vi "Log Plugin Errors.vi"(8 "error in (no error)":errorcluster, 11 "Full Plugin Array":T1[](array[typedef])) -> (0 "error out":errorcluster)   [LabVIEW 2020, in "RxnRover.lvlib" / "Plugin Manager.lvlib"]
doc: "This VI logs errors within invalid RxnRover plugins in a .txt file located at : \nwith the format;\n[Time RTC 3339] [Plugin name] Error : (error message) \n[Time RTC 3339] [Plugin name] Error : (error message) \n[Time RTC 3339] [Plugin name] Error : (error message) \n. . .\n\nIf there are no errors present, or invalid plugins, a .txt log file will not be created.\nlog file is overwritten at the standard path each time Load Plugins.vi is called (It does not create an additional log file)\nErrors are generated within the Read Configuration File .vi and sorted as invalid plugins within the Filter Invalid Plugins.vi\n\nCreated 5/20/2025 - Labview 2020\nRxnRover"
uses:
  Plugin Manager.lvlib
  Plugin Details.ctl
  Plugin Servers/Controller/Controller Type.ctl
  Plugin Types.ctl
  Config Error.ctl
  logging/logging.lvlib
  Plugin Servers/Controller/Generic Plugin.lvclass
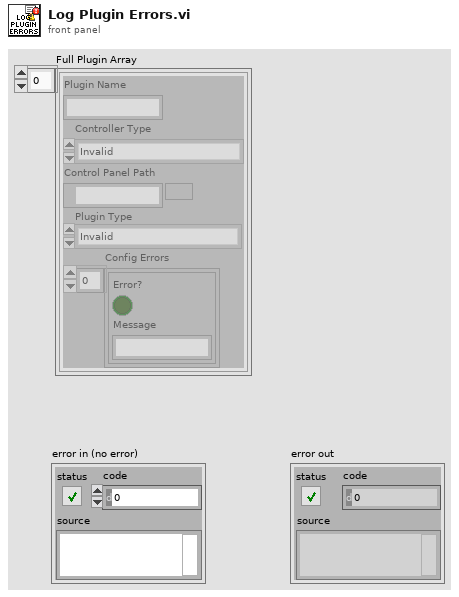
[diagram p1: front panel]
types:
  T1 = typedef "RxnRover.lvlib/Plugin Manager.lvlib/Plugin Details.ctl" = cluster{"Plugin Name":string, "Controller Type":T2, "Control Panel Path":path, "Plugin Type":T3, "Config Errors":T4[]}
  T2 = typedef "RxnRover.lvlib/Generic Plugin.lvclass/Controller Type.ctl" = enum16{"Invalid", "Temperature Controller", "Pump Controller", "Syringe Pump", "Generic Optimizer", "LC Parser", "Passive Hardware"}
  T3 = typedef "RxnRover.lvlib/Plugin Manager.lvlib/Plugin Types.ctl" = enum16{"Invalid", "Optimizer", "Analyzer", "Hardware"}
  T4 = typedef "RxnRover.lvlib/Plugin Manager.lvlib/Config Error.ctl" = cluster{"Error?":bool, "Message":string}
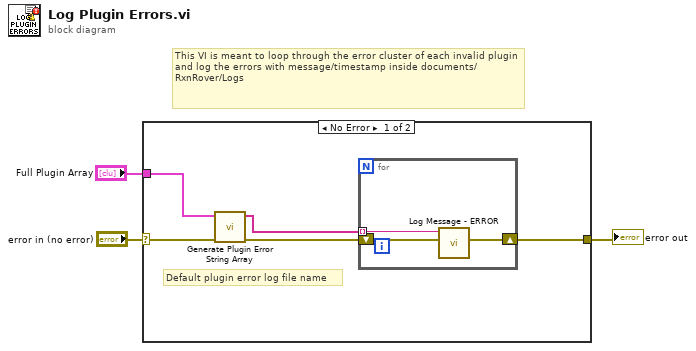
[diagram p0: block diagram]
diagram:
  # "This VI is meant to loop through the error cluster of each invalid plugin and log the errors with message/timestamp inside documents/RxnRover/Logs"
  n1 = case shown="No Error" "error in (no error)" {
    selector: "error in (no error)" -> [w5 w12]
    tunnel: "Full Plugin Array" -> [w8 _]
    tunnel: [w7 w12] -> w2
    frame No Error {
      # "Default plugin error log file name"
      n2 = call "Generate Plugin Error String Array.vi"("error in (no error)"=w5, "Full Plugin Array"=w8) -> ("error out"=w4:errorcluster, "Error Strings"=w6:string[])  [unwired: 8 in]
      n3 = for {
        shift-right: [w10] -> w7
        shift-left: w4 -> [w11]
        tunnel: w6 -> [w9] mode=indexing
        n4 = call "Log Message - ERROR.vi"("error in (no error)"=w11, "Message"=w9) -> ("error out"=w10:errorcluster)  [unwired: 9 in]
      }
    }
    frame Error {
    }
  }
  "error out" <- w2
